vi "PV Info Data from INI.vi"(8 "error in":errorcluster, 11 "Config Refnum in":T1) -> (0 "error out":errorcluster, 3 "Config Refnum out":T1, 4 "PV_Info":T2)   [LabVIEW 2017]
uses:
  <vilib>/Utility/config.llb/Config Data RefNum.ctl
  <vilib>/ORNL/CSEISMIC DDS/CSEISMIC DDS Base/Data Types/PV_Info.ctl
  <vilib>/ORNL/CSEISMIC DDS/CSEISMIC DDS Base/Data Types/Controls/DeviceID.ctl
  <vilib>/Utility/config.llb/Read Key (String).vi
  <vilib>/Utility/config.llb/Read Key (Double).vi
  <vilib>/Utility/config.llb/NI_LVConfig.lvlib
  <vilib>/ORNL/CSEISMIC DDS/CSEISMIC DDS Base/CSEISMIC DDS.lvclass
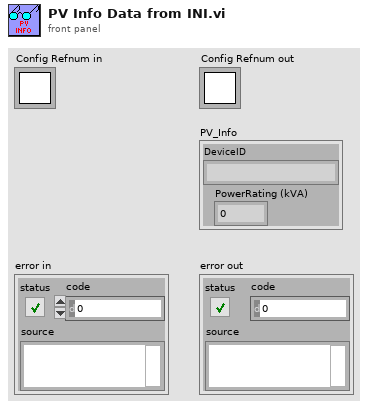
[diagram p1: front panel]
types:
  T1 = typedef "NI_LVConfig.lvlib/Config Data RefNum.ctl" = refnum<k1>
  T2 = typedef "CSEISMIC DDS.lvlib/CSEISMIC DDS.lvclass/PV_Info.ctl" = cluster{"DeviceID":T3, "PowerRating (kVA)":dbl}
  T3 = typedef "CSEISMIC DDS.lvlib/CSEISMIC DDS.lvclass/DeviceID.ctl" = string
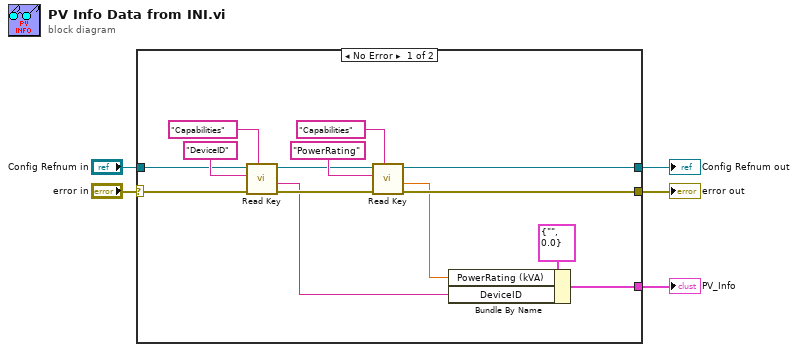
[diagram p0: block diagram]
diagram:
  n1 = case shown="No Error" "error in" {
    selector: "error in" -> [w7 w21]
    tunnel: [w19 w21] -> w5
    tunnel: [w18 w20] -> w4
    tunnel: [w17 _] -> w3
    tunnel: "Config Refnum in" -> [w8 w20]
    frame No Error {
      n2 = call-poly <vilib>:"Read Key.vi"("section"="Capabilities", "error in (no error)"=w7, "key"="DeviceID", "refnum"=w8) -> ("error out"=w9:errorcluster, "value"=w6:string, "refnum out"=w10:T1)  [unwired: 4 in, 1 out]
      n3 = call-poly <vilib>:"Read Key.vi"("section"="Capabilities", "error in (no error)"=w9, "key"="PowerRating", "refnum"=w10) -> ("error out"=w19:errorcluster, "value"=w16:dbl, "refnum out"=w18:T1)  [unwired: 4 in, 1 out]
      n4 = Bundle By Name(cluster=T2 {"DeviceID"="", "PowerRating (kVA)"=0.0} ("PV_Info"), "PowerRating (kVA)"=w16, "DeviceID"=w6) -> (w17:T2)
    }
    frame Error {
    }
  }
  "error out" <- w5
  "Config Refnum out" <- w4
  "PV_Info" <- w3
